vi "Drive_Loop_Control_Loop.vi"(4 "Priority\n- Specifies the priority of execution of the next frame relative\nto other timed events.\nMust be -1 or an integer between 1 & 65,535. \nDefault is -1 which means priority is unchanged\nfrom previous frame.":i32=100, 6 "Period \n- Amount of time between iterations of the timed control loop":i64=20, 7 "PID Gains":T1, 10 "RobotDriveDevRef":T2, 11 "Control Cluster":T10) -> ()   [LabVIEW 2015]
doc: "Help file written by FRC Team 836 - The RoboBees\n\nThis VI combines movment commands with various sensor inputs to control the robot as desired.\n\nThis VI uses VIs & Controls from Worcestor Polytechnic Institure (WPI) located in folder:\nC:\\Program Files (x86)\\National Instruments\\LabVIEW 2015\\vi.lib\\Rock Robotics\\WPI\\RobotDrive\n\nThe RobotDrive VI from WPI does the actual moving of the robot. The RobotDriveDevRef control\nwill pass commands to the WPI VI \"WPI_RobotDriveMotors\" via the WPI VI \"WPI_RobotDriveTankDrive\" to acutate the motors.\n\nThe RT FIFOs must be initialized using the \"Drive_Loop_Initialize_w_Help\" VI."
uses:
  <userlib>/836-Library/Drive/Drive_Code/Drive_Code_Support/Drive_Code_Bundle.ctl
  <userlib>/836-Library/Drive/Drive_Code/Drive_Code_Support/Sensor_Cluster.ctl
  <userlib>/836-Library/Drive/Drive_Code/Drive_Code_Support/Camera_Cluster.ctl
  <userlib>/836-Library/Drive/Drive_Code/Drive_Code_Support/Drive_Code_Notifier.ctl
  <userlib>/836-Library/Drive/Drive_Code/Drive_Code_Support/Drive_Code_Command.ctl
  <userlib>/836-Library/Drive/Drive_Code/Logging_Data.ctl
  <vilib>/Rock Robotics/WPI/RobotDrive/WPI_RobotDriveDevRef.ctl
  <vilib>/Rock Robotics/WPI/MotorControl/WPI_MotorControlDeviceRef.ctl
  <vilib>/Rock Robotics/WPI/MotorControl/WPI_MotorControlType.ctl
  <vilib>/Rock Robotics/SystemInterfaces/DIO/FPGA_DIOPWMChannel.ctl
  <vilib>/Rock Robotics/WPI/PWM/WPI_PWMDeadband.ctl
  <vilib>/Rock Robotics/WPI/CAN/Jaguar/SubVIs/WPI_CANJaguar_ControlMode.ctl
  <vilib>/Rock Robotics/WPI/CAN/TalonSRX/WPI_CANTalonSRX_APIControlMode.ctl
  <userlib>/836-Library/Drive/Drive_Code/Drive_Code_Support/Drive_Code_PID_Bundle.ctl
  <vilib>/Platform/TimedLoop/XDataNode/timing_clust.ctl
  <vilib>/Platform/TimedLoop/XDataNode/nitl_modes.ctl
  <vilib>/Platform/TimedLoop/XDataNode/wakeup.ctl
  <userlib>/836-Library/Drive/Drive_Code/Drive_Code_Support/Drive_Types.ctl
  <vilib>/addons/control/pid/pid.llb/PID (DBL).vi
  <vilib>/platform/TimedLoop/XDataNode/XDataNode.xnode
  <vilib>/Platform/TimedLoop/XDataNode/XDNodeRunTimeDep.lvlib
  <vilib>/addons/control/pid/NI_PID_pid.lvlib
panel:
  out "Right":dbl(graph)
  out "Left":dbl(graph)
  out "State":dbl(graph)
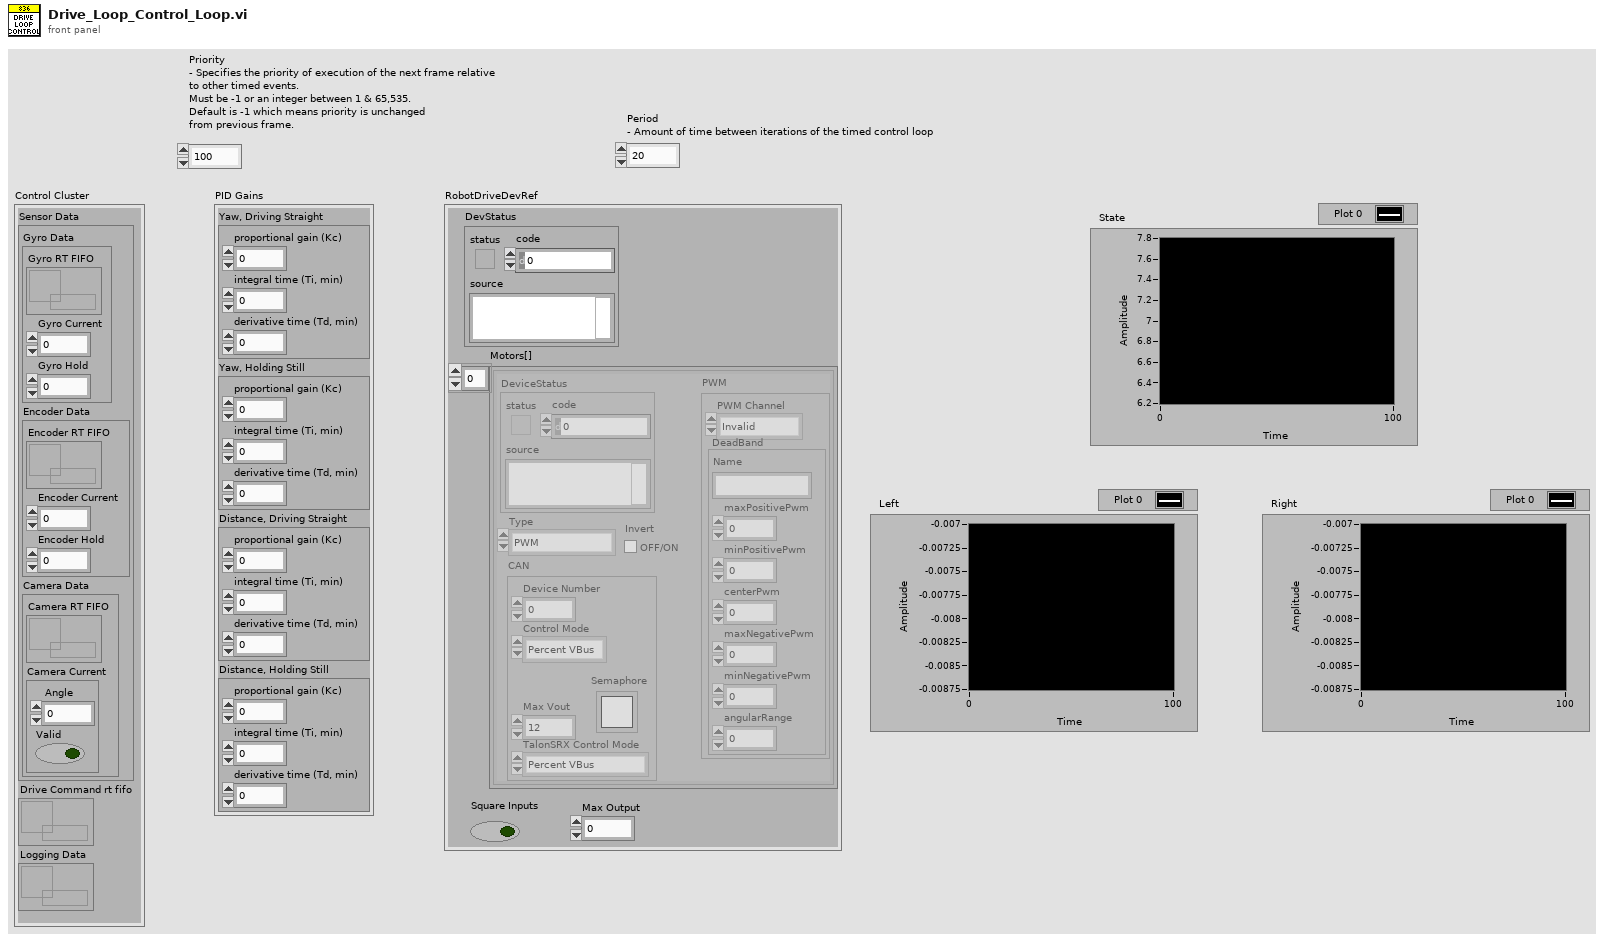
[diagram p1: front panel]
types:
  T1 = typedef "Drive_Code_PID_Bundle.ctl" = cluster{"Yaw, Driving Straight":cluster{"proportional gain (Kc)":dbl, "integral time (Ti, min)":dbl, "derivative time (Td, min)":dbl}, "Yaw, Holding Still":cluster{"proportional gain (Kc)":dbl, "integral time (Ti, min)":dbl, "derivative time (Td, min)":dbl}, "Distance, Driving Straight":cluster{"proportional gain (Kc)":dbl, "integral time (Ti, min)":dbl, "derivative time (Td, min)":dbl}, "Distance, Holding Still":cluster{"proportional gain (Kc)":dbl, "integral time (Ti, min)":dbl, "derivative time (Td, min)":dbl}}
  T2 = typedef "WPI_RobotDriveDevRef.ctl" = cluster{"DevStatus":errorcluster, "Motors[]":T3[], "Square Inputs":bool, "Max Output":dbl}
  T3 = typedef "WPI_MotorControlDeviceRef.ctl" = cluster{"DeviceStatus":errorcluster, "Type":T4, "PWM":cluster{"PWM Channel":T5, "DeadBand":T6}, "CAN":cluster{"Device Number":u8, "Control Mode":T7, "Semaphore":T8, "Max Vout":dbl, "TalonSRX Control Mode":T9}, "Invert":bool}
  T4 = typedef "WPI_MotorControlType.ctl" = enum16{"PWM", "CAN", "CANTalonSRX"}
  T5 = typedef "FPGA_DIOPWMChannel.ctl" = enum8{"PWM 0", "PWM 1", "PWM 2", "PWM 3", "PWM 4", "PWM 5", "PWM 6", "PWM 7", "PWM 8", "PWM 9", "PWM MXP 0", "PWM MXP 1", "PWM MXP 2", "PWM MXP 3", "PWM MXP 4", "PWM MXP 5", "PWM MXP 6", "PWM MXP 7", "PWM MXP 8", "PWM MXP 9", "Invalid"}
  T6 = typedef "WPI_PWMDeadband.ctl" = cluster{"Name":string, "maxPositivePwm":i32, "minPositivePwm":i32, "centerPwm":i32, "maxNegativePwm":i32, "minNegativePwm":i32, "angularRange":u16}
  T7 = typedef "WPI_CANJaguar_ControlMode.ctl" = enum8{"Percent VBus", "Current", "Speed", "Position", "Voltage"}
  T8 = typedef "Semaphore RefNum" = refnum<k1>
  T9 = typedef "WPI_CANTalonSRX_APIControlMode.ctl" = enum8{"Percent VBus", "Speed", "Position", "Slave", "Unchanged / Invalid", "Voltage Compensation", "Current", "Motion Profile"}
  T10 = typedef "Drive_Code_Bundle.ctl" = cluster{"Sensor Data":T11, "Drive Command rt fifo":refnum<k33>, "Logging Data":refnum<k33>}
  T11 = typedef "Sensor_Cluster.ctl" = cluster{"Gyro Data":cluster{"Gyro RT FIFO":refnum<k33>, "Gyro Current":dbl, "Gyro Hold":dbl}, "Encoder Data":cluster{"Encoder RT FIFO":refnum<k33>, "Encoder Current":dbl, "Encoder Hold":dbl}, "Camera Data":cluster{"Camera RT FIFO":refnum<k33>, "Camera Current":T12}}
  T12 = typedef "Camera_Cluster.ctl" = cluster{" Angle":dbl, "Valid":bool}
  T13 = typedef "Logging_Data.ctl" = cluster{"Command":T14, "Desired Angle":dbl, "Desired Encoder":dbl}
  T14 = typedef "Drive_Code_Command.ctl" = enum16{"Do Nothing", "Manual", "Drive Continuous", "Turn", "Drive Distance", "Hold Position", "Hold Yaw", "Follow Camera", "Turn to Camera"}
  T15 = typedef "Drive_Code_Notifier.ctl" = cluster{"Command":T14, "Parameter A":dbl, "Parameter B":dbl, "Parameter C":dbl, "Absolute?":bool}
  T16 = typedef "XDNodeRunTimeDep.lvlib/timing_clust.ctl" = cluster{"Expected End [f-1]":u64, "Actual End [f-1]":u64, "Finished Late? [f-1]":bool, "Expected End [i-1]":u64, "Actual End [i-1]":u64, "Finished Late? [i-1]":bool, "Expected Start [i]":u64, "Actual Start [i]":u64, "Expected Start [f]":u64, "Actual Start [f]":u64, "Source Name":string, "Structure Name":string, "Period":i64, "Deadline":i64, "Offset":i64, "Start":i64, "Priority":i32, "Timeout":i32, "Mode":T17, "Wakeup Reason":T18, "Error":errorcluster, "Source Type":string, "Secondary Source Type":string, "Global End Time":u64, "Global Start Time":u64, "Frame Duration":u64, "Iteration Duration":u64, "Assigned CPU":i32, "I/O Scan Engine Mode":u32}
  T17 = typedef "XDNodeRunTimeDep.lvlib/nitl_modes.ctl" = enum32{"No Change", "Process missed periods, maintain original phase", "Discard missed periods, maintain original phase", "Process missed periods, ignore original phase", "Discard missed periods, ignore original phase"}
  T18 = typedef "XDNodeRunTimeDep.lvlib/wakeup.ctl" = enum32{"Normal", "Aborted", "Asynchronous wakeup", "Timing source error", "Timed loop error", "Timeout"}
  T19 = typedef "Drive_Types.ctl" = enum16{"Tank Drive", "Cheesy Drive Yaw PID", "Cheesy Drive Full PID"}
  T20 = cluster{"Gyro RT FIFO":refnum<k33>, "Gyro Current":dbl, "Gyro Hold":dbl}
  T21 = cluster{"Encoder RT FIFO":refnum<k33>, "Encoder Current":dbl, "Encoder Hold":dbl}
  T22 = cluster{"Camera RT FIFO":refnum<k33>, "Camera Current":T12}
  T23 = cluster{"proportional gain (Kc)":dbl, "integral time (Ti, min)":dbl, "derivative time (Td, min)":dbl}
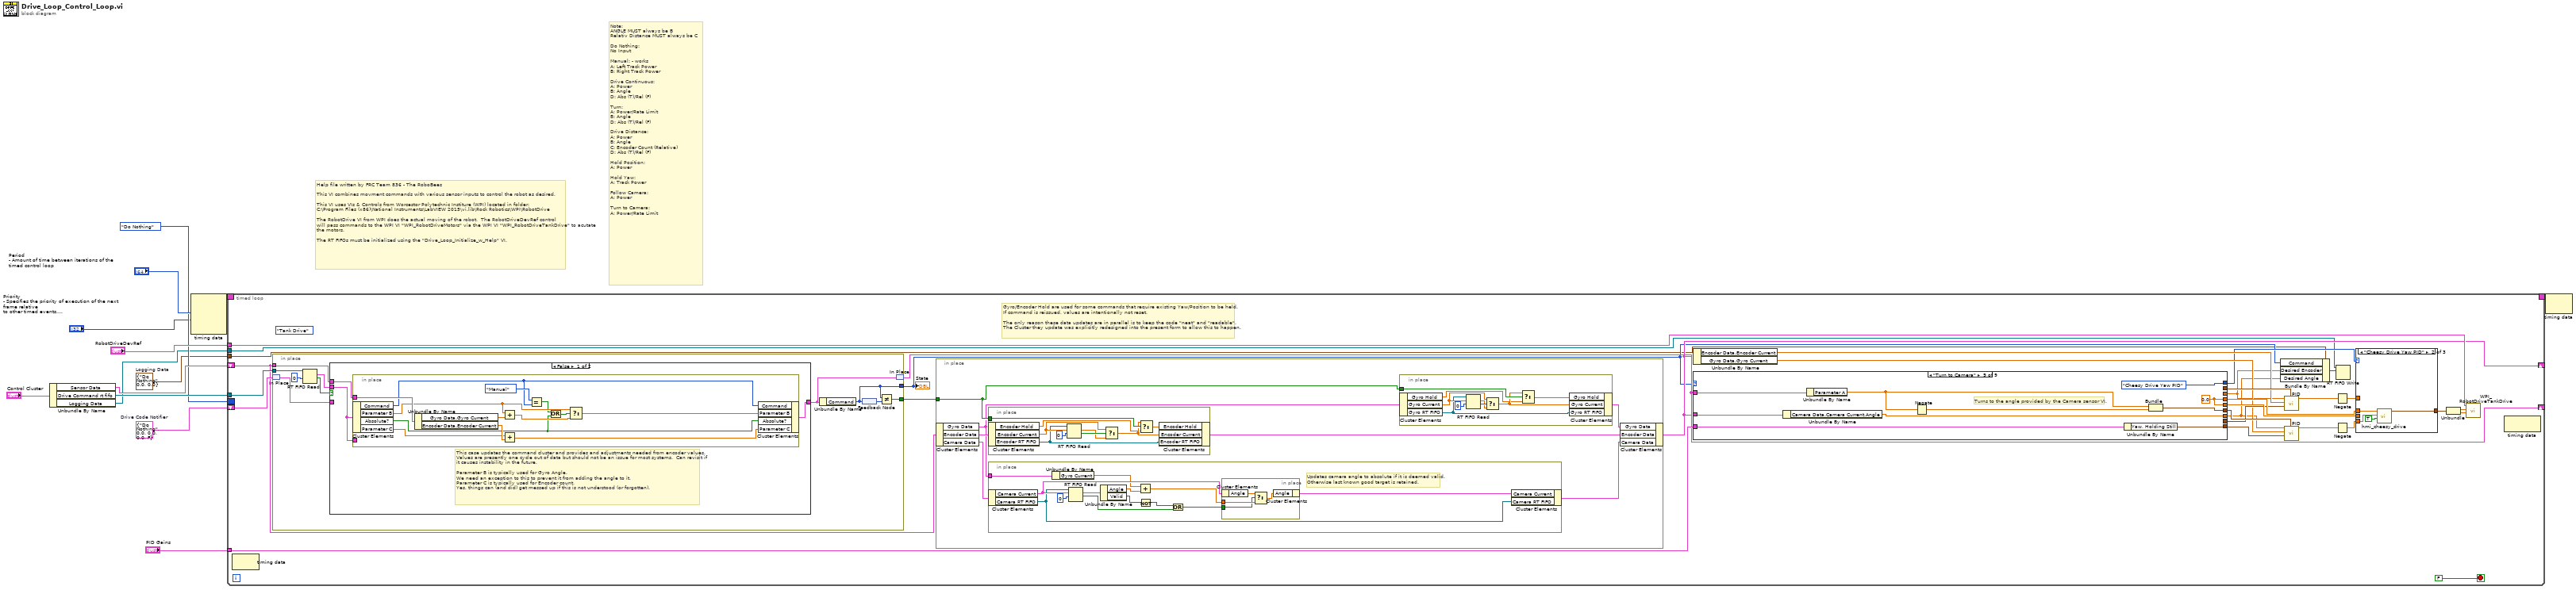
[diagram p0: block diagram]
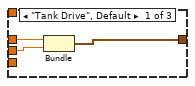
[diagram p3: hidden frame]
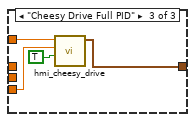
[diagram p4: hidden frame]
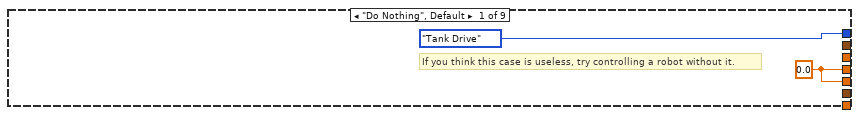
[diagram p5: hidden frame]
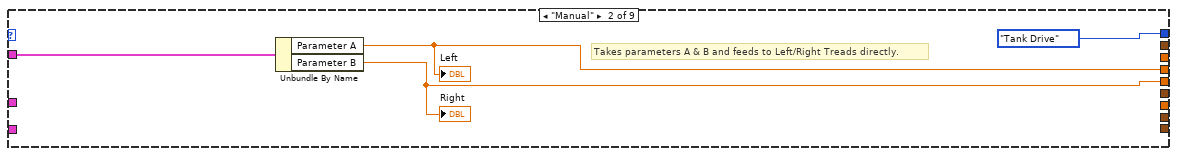
[diagram p6: hidden frame]
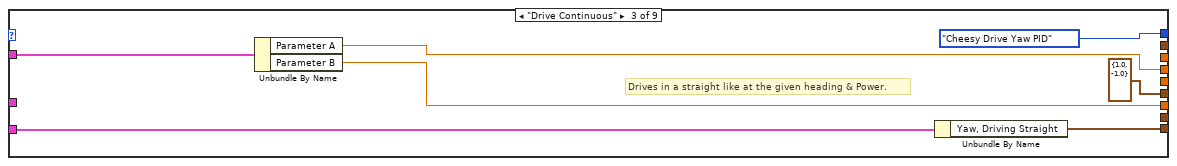
[diagram p7: hidden frame]
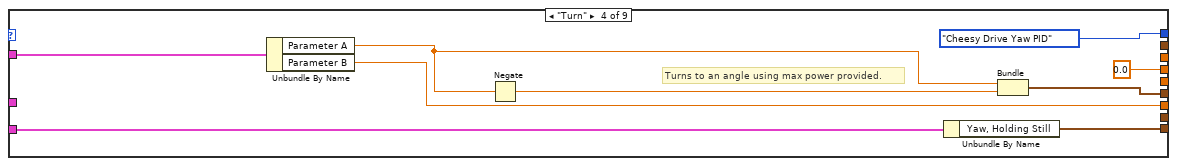
[diagram p8: hidden frame]
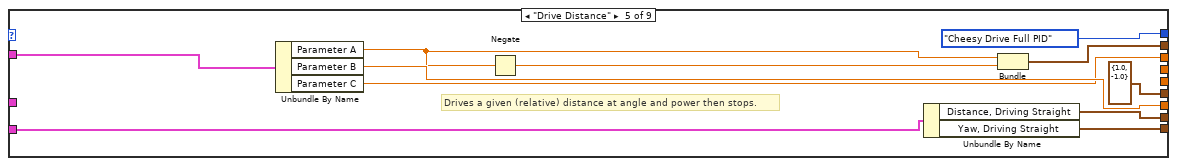
[diagram p9: hidden frame]
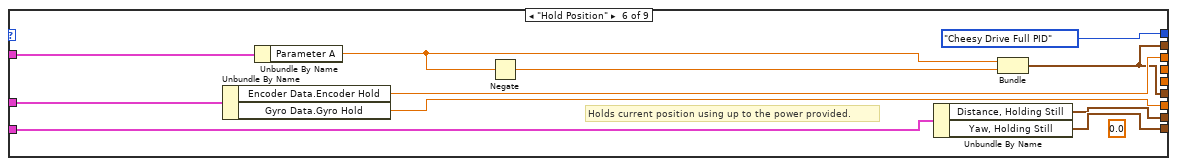
[diagram p10: hidden frame]
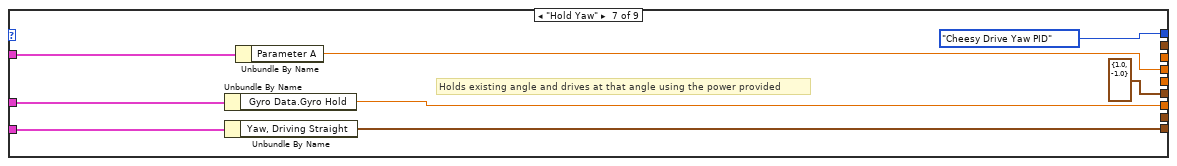
[diagram p11: hidden frame]
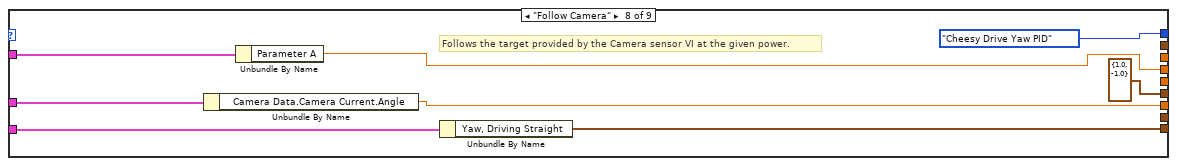
[diagram p12: hidden frame]
diagram:
  w1 = T13 {"Command"=enum."Do Nothing", "Desired Angle"=0.0, "Desired Encoder"=0.0}  # Logging Data
  w4 = T15 {"Command"=enum."Do Nothing", "Parameter A"=0.0, "Parameter B"=0.0, "Parameter C"=0.0, "Absolute?"=FALSE}  # Drive Code Notifier
  # "Help file written by FRC Team 836 - The RoboBees\n\nThis VI combines movment commands with various sensor inputs to control the robot as desired.\n\nThis VI uses VIs & Controls from Worcestor Polytechnic Institure (WPI) located in folder:\nC:\\Program Files (x86)\\National Instruments\\LabVIEW 2015\\vi.lib\\Rock Robotics\\WPI\\RobotDrive\n\nThe RobotDrive VI from WPI does the actual moving of the robot.  The RobotDriveDevRef control\nwill pass commands to the WPI VI \"WPI_RobotDriveMotors\" via the WPI VI \"WPI_RobotDriveTankDrive\" to acutate the motors.\n\nThe RT FIFOs must be initialized using the \"Drive_Loop_Initialize_w_Help\" VI."
  # "Note:  \nANGLE MUST always be B\nRelativ Distance MUST always be C\n\nDo Nothing:\nNo Input\n\nManual: - works\nA: Left Track Power\nB: Right Track Power\n\nDrive Continuous:\nA: Power\nB: Angle\nD: Abs (T)/Rel (F)\n\nTurn:\nA: Power/Rate Limit\nB: Angle\nD: Abs (T)/Rel (F)\n\nDrive Distance:\nA: Power\nB: Angle\nC: Encoder Count (Relative)\nD: Abs (T)/Rel (F)\n\nHold Position:\nA: Power\n\nHold Yaw:\nA: Track Power\n\nFollow Camera:\nA: Power\n\nTurn to Camera:\nA: Power/Rate Limit"
  n1 = Unbundle By Name("Control Cluster") -> ("Sensor Data"=w11:T11, "Drive Command rt fifo"=w10:refnum<k33>, "Logging Data"=w2:refnum<k33>)
  n2 = node-c288("Period \n- Amount of time between iterations of the timed control loop", "Priority\n- Specifies the priority of execution of the next frame relative\nto other timed events.\nMust be -1 or an integer between 1 & 65,535. \nDefault is -1 which means priority is unchanged\nfrom previous frame.") -> (w13:T16)  [unwired: 2 in]
  n3 = timed-loop {
    timing: w13 -> [_]
    timing-out: [_] -> w12
    shift-right: [w25] -> _
    shift-left: w4 -> [w26]
    tunnel: "PID Gains" -> [w43]
    tunnel: "RobotDriveDevRef" -> [w31]
    tunnel: w10 -> [w30]
    border: Drive_Code_Command."Do Nothing" ("Command") -> [_]
    shift-right: [w24] -> _
    shift-left: w11 -> [w20]
    tunnel: w2 -> [w19]
    tunnel: w1 -> [w14]
    stop <- FALSE stop-if-true
    (unwired) Drive_Types."Tank Drive"
    # "Gyro/Encoder Hold are used for some commands that require existing Yaw/Position to be held.\nIf command is reissued, values are intentionally not reset.\n\nThe only reason these data updates are in parallel is to keep the code \"neat\" and \"readable\".\nThe Cluster they update was explicitly redesigned into the present form to allow this to happen."
    n4 = node-c288() -> ()  [unwired: 1 in, 1 out]
    n5 = in-place {
      in-place-border: w30 -> [w96]
      in-place-border: [w93] -> w29
      in-place-border: [w92] -> w17
      in-place-border: w20 -> [w90]
      n6 = in-place-match #1(w26) -> (w88:T15)
      n7 = RT FIFO Read(0:w96, 2:0 ("timeout in ms (0)")) -> (9:w91:T15, 10:w89:bool)  [unwired: 2 in, 3 out]
      n8 = case shown="False" w89 {
        tunnel: w91 -> [w98 _]
        tunnel: [w97 w113] -> w87
        tunnel: w90 -> [w99 _]
        tunnel: w88 -> [_ w113]
        frame False {
          # "This case updates the command cluster and provides and adjustments needed from encoder values.\nValues are presently one cycle out of data but should not be an issue for most systems.  Can revisit if\nit causes instability in the future.\n\nParameter B is typically used for Gyro Angle.  \nWe need an exception to this to prevent it from adding the angle to it.\nParameter C is typically used for Encoder count. \nYes, things can (and did) get messed up if this is not understood (or forgotten)."
          n9 = in-place {
            in-place-border: w98 -> [_]
            in-place-border: w99 -> [w111]
            n10 = in-place-cluster #2(w98) -> ("Command"=w100:T14, "Parameter B"=w108:dbl, "Absolute?"=w102:bool, "Parameter C"=w106:dbl)
            n11 = Unbundle By Name(w111) -> ("Gyro Data.Gyro Current"=w110:dbl, "Encoder Data.Encoder Current"=w109:dbl)
            n12 = Add(x=w108, y=w110) -> (x+y=w112:dbl)
            n13 = Add(x=w106, y=w109) -> (x+y=w105:dbl)
            n14 = Equal?(x=Drive_Code_Command."Manual" ("Command"), y=w100) -> (x = y?=w103:bool)
            n15 = Or(x=w103, y=w102) -> (x .or. y?=w101:bool)
            n16 = Select(t=w108, s=w101, f=w112) -> (s? t:f=w107:dbl)
            n17 = in-place-cluster #2("Command"=w100, "Parameter B"=w107, "Absolute?"=w102, "Parameter C"=w105) -> (w97:T15)
          }
        }
        frame True {
          # "Timeout case, no update to command loop."
        }
      }
      n18 = Unbundle By Name(w87) -> ("Command"=w92:T14)
      n19 = feedback #3() -> (w94:T14)
      n20 = feedback-in #3(w92) -> ()
      n21 = Not Equal?(x=w92, y=w94) -> (x != y?=w93:bool)
      n22 = in-place-match #1(w87) -> (w25:T15)
    }
    "State" <- w17
    n23 = in-place {
      in-place-border: w29 -> [w46]
      n24 = in-place-cluster #4(w20) -> ("Gyro Data"=w45:T20, "Encoder Data"=w50:T21, "Camera Data"=w48:T22)
      n25 = in-place {
        in-place-border: w46 -> [w75]
        n26 = in-place-cluster #5(w50) -> ("Encoder Hold"=w73:dbl, "Encoder Current"=w71:dbl, "Encoder RT FIFO"=w69:refnum<k33>)
        n27 = RT FIFO Read(0:w69, 1:w71, 2:0 ("timeout in ms (0)")) -> (9:w76:dbl, 10:w77:bool)  [unwired: 1 in, 3 out]
        n28 = Select(t=w71, s=w77, f=w76) -> (s? t:f=w74:dbl)
        n29 = Select(t=w74, s=w75, f=w73) -> (s? t:f=w72:dbl)
        n30 = in-place-cluster #5("Encoder Hold"=w72, "Encoder Current"=w74, "Encoder RT FIFO"=w69) -> (w49:T21)
      }
      n31 = in-place {
        in-place-border: w45 -> [w53]
        # "Updates camera angle to absolute if it is deemed valid.\nOtherwise last known good target is retained."
        n32 = in-place-cluster #6(w48) -> ("Camera Current"=w55:T12, "Camera RT FIFO"=w54:refnum<k33>)
        n33 = Unbundle By Name(w53) -> ("Gyro Current"=w52:dbl)
        n34 = RT FIFO Read(0:w54, 1:w55, 2:0 ("timeout in ms (0)")) -> (9:w64:T12, 10:w60:bool)  [unwired: 1 in, 3 out]
        n35 = Unbundle By Name(w64) -> ("Angle"=w63:dbl, "Valid"=w61:bool)
        n36 = Add(x=w52, y=w63) -> (x+y=w62:dbl)
        n37 = Not(x=w61) -> (.not. x?=w58:bool)
        n38 = Or(x=w58, y=w60) -> (x .or. y?=w59:bool)
        n39 = in-place {
          in-place-border: w62 -> [w68]
          in-place-border: w59 -> [w67]
          n40 = in-place-cluster #7(w55) -> ("Angle"=w66:dbl)
          n41 = Select(t=w66, s=w67, f=w68) -> (s? t:f=w65:dbl)
          n42 = in-place-cluster #7("Angle"=w65) -> (w56:T12)
        }
        n43 = in-place-cluster #6("Camera Current"=w56, "Camera RT FIFO"=w54) -> (w47:T22)
      }
      n44 = in-place {
        in-place-border: w46 -> [w84]
        n45 = in-place-cluster #8(w45) -> ("Gyro Hold"=w81:dbl, "Gyro Current"=w80:dbl, "Gyro RT FIFO"=w78:refnum<k33>)
        n46 = RT FIFO Read(0:w78, 1:w80, 2:0 ("timeout in ms (0)")) -> (9:w85:dbl, 10:w86:bool)  [unwired: 1 in, 3 out]
        n47 = Select(t=w80, s=w86, f=w85) -> (s? t:f=w83:dbl)
        n48 = Select(t=w83, s=w84, f=w81) -> (s? t:f=w82:dbl)
        n49 = in-place-cluster #8("Gyro Hold"=w82, "Gyro Current"=w83, "Gyro RT FIFO"=w78) -> (w51:T20)
      }
      n50 = in-place-cluster #4("Gyro Data"=w51, "Encoder Data"=w49, "Camera Data"=w47) -> (w24:T11)
    }
    n51 = Unbundle By Name(w24) -> ("Encoder Data.Encoder Current"=w27:dbl, "Gyro Data.Gyro Current"=w28:dbl)
    n52 = case shown="\"Turn to Camera\"" w17 {
      tunnel: w43 -> [_ _ w134 w140 w151 w168 w174 w182 w194]
      tunnel: w25 -> [_ w130 w137 w146 w157 w165 w176 w184 w192]
      tunnel: [w126 w128 w136 0.0 ("Parameter A") _ _ w175 w183 w188] -> w42
      tunnel: [w126 w127 _ _ _ _ _ _ w188] -> w41
      tunnel: [_ _ w135 w141 w156 w160 w171 w179 w186] -> w15
      tunnel: [_ _ w133 w139 w149 w167 w173 w181 w193] -> w39
      tunnel: [_ _ cluster{"output high":dbl, "output low":dbl} {"output high"=1.0, "output low"=-1.0} ("output range") w142 cluster{"Parameter A":dbl, "output low":dbl} {"Parameter A"=1.0, "output low"=-1.0} ("output range") w158 cluster{"Parameter A":dbl, "output low":dbl} {"Parameter A"=1.0, "output low"=-1.0} ("output range") cluster{"Parameter A":dbl, "output low":dbl} {"Parameter A"=1.0, "output low"=-1.0} ("output range") w189] -> w38
      tunnel: [_ _ _ _ w155 w161 _ _ _] -> w16
      tunnel: [_ _ _ _ w152 w158 _ _ _] -> w33
      tunnel: [_ _ _ _ w150 w166 _ _ _] -> w32
      tunnel: w24 -> [_ _ _ _ _ w162 w172 w180 w187]
      tunnel: [Drive_Types."Tank Drive" Drive_Types."Tank Drive" Drive_Types."Cheesy Drive Yaw PID" Drive_Types."Cheesy Drive Yaw PID" Drive_Types."Cheesy Drive Full PID" Drive_Types."Cheesy Drive Full PID" Drive_Types."Cheesy Drive Yaw PID" Drive_Types."Cheesy Drive Yaw PID" Drive_Types."Cheesy Drive Yaw PID"] -> w23
      frame "Do Nothing", Default {
        w126 = 0.0 ("Parameter A")
        # "If you think this case is useless, try controlling a robot without it."
      }
      frame "Manual" {
        # "Takes parameters A & B and feeds to Left/Right Treads directly."
        n53 = Unbundle By Name(w130) -> ("Parameter A"=w128:dbl, "Parameter B"=w127:dbl)
        "Left" <- w128
        "Right" <- w127
      }
      frame "Drive Continuous" {
        # "Drives in a straight like at the given heading & Power."
        n54 = Unbundle By Name(w137) -> ("Parameter A"=w136:dbl, "Parameter B"=w135:dbl)
        n55 = Unbundle By Name(w134) -> ("Yaw, Driving Straight"=w133:T23)
      }
      frame "Turn" {
        # "Turns to an angle using max power provided."
        n56 = Unbundle By Name(w146) -> ("Parameter A"=w144:dbl, "Parameter B"=w141:dbl)
        n57 = Negate(x=w144) -> (-x=w143:dbl)
        n58 = Unbundle By Name(w140) -> ("Yaw, Holding Still"=w139:T23)
        n59 = Bundle("Parameter A"=w144, w143) -> (w142:cluster{"Parameter A":dbl, dbl})  [unwired: 1 in]
      }
      frame "Drive Distance" {
        # "Drives a given (relative) distance at angle and power then stops."
        n60 = Unbundle By Name(w157) -> ("Parameter A"=w153:dbl, "Parameter B"=w156:dbl, "Parameter C"=w155:dbl)
        n61 = Negate(x=w153) -> (-x=w154:dbl)
        n62 = Unbundle By Name(w151) -> ("Distance, Driving Straight"=w150:T23, "Yaw, Driving Straight"=w149:T23)
        n63 = Bundle("Parameter A"=w153, w154) -> (w152:cluster{"Parameter A":dbl, dbl})  [unwired: 1 in]
      }
      frame "Hold Position" {
        (unwired) 0.0 ("Encoder Data.Encoder Hold")
        # "Holds current position using up to the power provided."
        n64 = Unbundle By Name(w162) -> ("Encoder Data.Encoder Hold"=w161:dbl, "Gyro Data.Gyro Hold"=w160:dbl)
        n65 = Unbundle By Name(w165) -> ("Parameter A"=w163:dbl)
        n66 = Negate(x=w163) -> (-x=w164:dbl)
        n67 = Unbundle By Name(w168) -> ("Distance, Holding Still"=w166:T23, "Yaw, Holding Still"=w167:T23)
        n68 = Bundle("Parameter A"=w163, w164) -> (w158:cluster{"Parameter A":dbl, dbl})  [unwired: 1 in]
      }
      frame "Hold Yaw" {
        # "Holds existing angle and drives at that angle using the power provided"
        n69 = Unbundle By Name(w172) -> ("Gyro Data.Gyro Hold"=w171:dbl)
        n70 = Unbundle By Name(w174) -> ("Yaw, Driving Straight"=w173:T23)
        n71 = Unbundle By Name(w176) -> ("Parameter A"=w175:dbl)
      }
      frame "Follow Camera" {
        # "Follows the target provided by the Camera sensor VI at the given power."
        n72 = Unbundle By Name(w180) -> ("Camera Data.Camera Current.Angle"=w179:dbl)
        n73 = Unbundle By Name(w184) -> ("Parameter A"=w183:dbl)
        n74 = Unbundle By Name(w182) -> ("Yaw, Driving Straight"=w181:T23)
      }
      frame "Turn to Camera" {
        w188 = 0.0 ("Parameter A")
        # "Turns to the angle provided by the Camera sensor VI."
        n75 = Unbundle By Name(w187) -> ("Camera Data.Camera Current.Angle"=w186:dbl)
        n76 = Unbundle By Name(w192) -> ("Parameter A"=w190:dbl)
        n77 = Negate(x=w190) -> (-x=w191:dbl)
        n78 = Unbundle By Name(w194) -> ("Yaw, Holding Still"=w193:T23)
        n79 = Bundle("Parameter A"=w190, w191) -> (w189:cluster{"Parameter A":dbl, dbl})  [unwired: 1 in]
      }
    }
    n80 = Bundle By Name(cluster=w14, "Command"=w17, "Desired Encoder"=w16, "Desired Angle"=w15) -> (w18:T13)
    n81 = call-poly <vilib>:"PID.vi"("output range"=w33, "PID gains"=w32, "process variable"=w27, "setpoint"=w16) -> ("output"=w34:dbl)  [unwired: 6 in, 1 out]
    n82 = call-poly <vilib>:"PID.vi"("output range"=w38, "PID gains"=w39, "process variable"=w28, "setpoint"=w15) -> ("output"=w40:dbl)  [unwired: 6 in, 1 out]
    n83 = Negate(x=w34) -> (-x=w21:dbl)
    n84 = Negate(x=w40) -> (-x=w22:dbl)
    n85 = RT FIFO Write(0:w19, 1:w18) -> ()  [unwired: 3 in, 4 out]
    n86 = case shown="\"Cheesy Drive Yaw PID\"" w23 {
      tunnel: w42 -> [w116 w119 _]
      tunnel: w41 -> [w115 _ _]
      tunnel: w22 -> [_ w120 w124]
      tunnel: [w114 w117 w122] -> w37
      tunnel: w21 -> [_ _ w121]
      frame "Tank Drive", Default {
        n87 = Bundle("Parameter A"=w116, "Parameter A"=w115) -> (w114:cluster{"Parameter A":dbl, "Parameter A":dbl})  [unwired: 1 in]
      }
      frame "Cheesy Drive Yaw PID" {
        n88 = call <userlib>:"hmi_cheesy_drive.vi"("Quick Turn"=TRUE, "Wheel"=w120, "Throttle"=w119) -> ("Drive Data"=w117:cluster{"Left":dbl, "Right":dbl})  [unwired: 8 in]
      }
      frame "Cheesy Drive Full PID" {
        n89 = call <userlib>:"hmi_cheesy_drive.vi"("Quick Turn"=TRUE, "Wheel"=w124, "Throttle"=w121) -> ("Drive Data"=w122:cluster{"Left":dbl, "Right":dbl})  [unwired: 8 in]
      }
    }
    n90 = Unbundle(w37) -> ("Left"=w36:dbl, "Right"=w35:dbl)
    n91 = call <vilib>:"WPI_RobotDriveTankDrive.vi"("Right axis value"=w35, "Left axis value"=w36, "RobotDriveDevRef"=w31) -> ()  [unwired: 6 in, 3 out]
    n92 = node-c288() -> ()  [unwired: 1 in, 1 out]
  }
  n93 = node-c288(w12) -> ()  [unwired: 1 out]
